vi "Write Configuration File from User.vi"(7 "Master?":bool=TRUE, 8 "error in":errorcluster, 10 "Master Config":T1 {"Conc Tolerance" min=0.0 max=100.0 step=1.0}, 11 "Test Config":T3={"Chopper RPM"=140, "IR Power"=5, "Conc Tolerance"=0.0, "Gas Stable Time"=0, "A-D Settle"=0, "Samples"=0, "Filter Time"=0, "Gas Mixtures"=[], "Filter Sequences"=[], "Functional Test"={"Mic Test ON ADC Max"=0.0, "Mic Test ON ADC Min"=0.0, "Mic Test OFF ADC Max"=0.0, "Mic Test OFF ADC Min"=0.0, "Mic Test IC ADC Max"=0.0, "Mic Test IC ADC Min"=0.0, "IR Emitter ON ADC Max"=0.0, "IR Emitter ON ADC Min"=0.0, "IR Emitter OFF ADC Max"=0.0, "IR Emitter OFF ADC Min"=0.0}, "Initial Flow Rate"=0.0, "Max Flow Rate"=0.0} {"Gas Mixtures"."ADC Gains" items=["0"=0, "3"=3, "4"=4, "5"=5, "6"=6, "7"=7]; "Conc Tolerance" min=0.0 max=100.0 step=1.0; "IR Power" min=2 max=5 step=1; "Chopper RPM" min=140 max=1000 step=1}) -> (0 "error out":errorcluster, 3 "Cancelled?":bool)   [LabVIEW 2015]
uses:
  Controls/Test Config.ctl
  Controls/Gas Mixture.ctl
  CAN Communication/PAS/Typedefs/ADC Gains.ctl
  Controls/Filter Sequence.ctl
  Controls/Functional Test.ctl
  Controls/Master Config.ctl
  Controls/Gas Info.ctl
  CAN Communication/PAS/PAS.lvclass
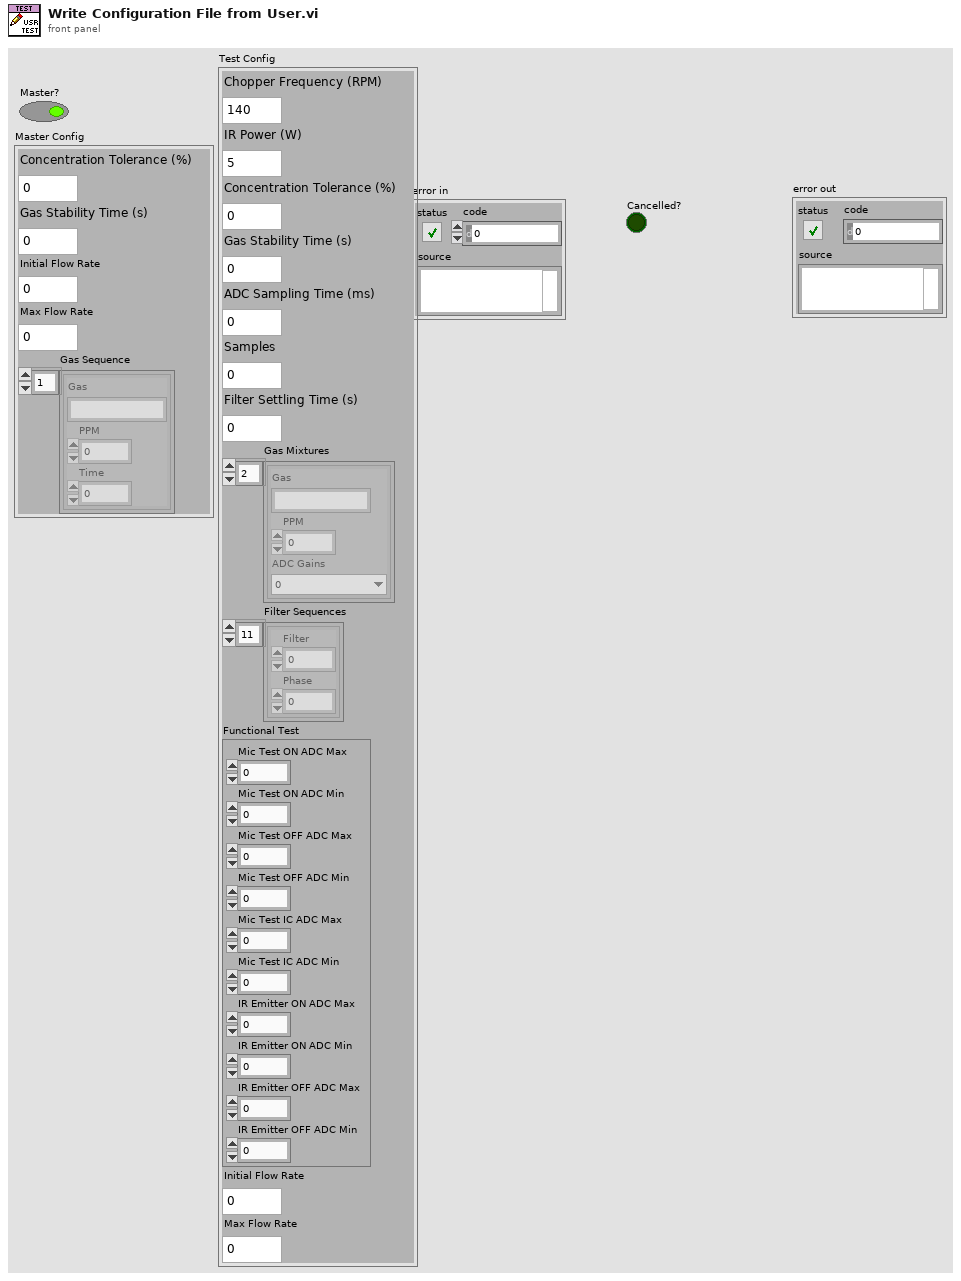
[diagram p1: front panel]
types:
  T1 = typedef "Master Config.ctl" = cluster{"Conc Tolerance":dbl, "Gas Stable Time":u16, "Initial Flow Rate":sgl, "Max Flow Rate":sgl, "Gas Sequence":T2[]}
  T2 = typedef "Gas Info.ctl" = cluster{"Gas":string, "PPM":dbl, "Time":u32}
  T3 = typedef "Test Config.ctl" = cluster{"Chopper RPM":u16, "IR Power":u8, "Conc Tolerance":dbl, "Gas Stable Time":u16, "A-D Settle":u16, "Samples":u16, "Filter Time":u16, "Gas Mixtures":T4[], "Filter Sequences":T6[], "Functional Test":T7, "Initial Flow Rate":sgl, "Max Flow Rate":sgl}
  T4 = typedef "Gas Mixture.ctl" = cluster{"Gas":string, "PPM":dbl, "ADC Gains":T5}
  T5 = typedef "PAS.lvclass/ADC Gains.ctl" = u16
  T6 = typedef "Filter Sequence.ctl" = cluster{"Filter":u8, "Phase":dbl}
  T7 = typedef "Functional Test.ctl" = cluster{"Mic Test ON ADC Max":dbl, "Mic Test ON ADC Min":dbl, "Mic Test OFF ADC Max":dbl, "Mic Test OFF ADC Min":dbl, "Mic Test IC ADC Max":dbl, "Mic Test IC ADC Min":dbl, "IR Emitter ON ADC Max":dbl, "IR Emitter ON ADC Min":dbl, "IR Emitter OFF ADC Max":dbl, "IR Emitter OFF ADC Min":dbl}
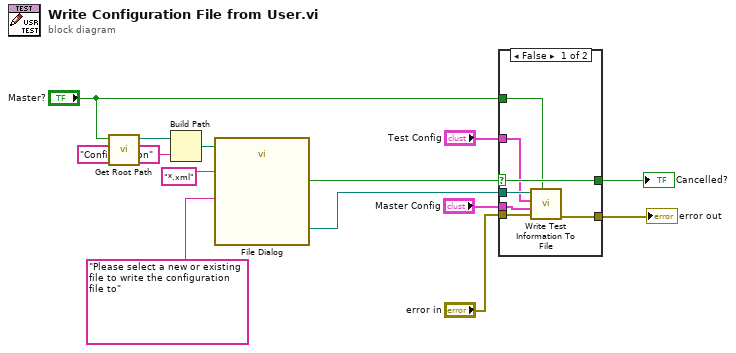
[diagram p0: block diagram]
diagram:
  n1 = call "Get Root Path.vi"("Master?"="Master?") -> ("Root Path"=w12:path)  [unwired: 10 in]
  n2 = Build Path(base path=w12, name or relative path="Configuration") -> (appended path=w11:path)
  n3 = call "File Dialog"("start path"=w11, "prompt"="Please select a new or existing file to write the configuration file to", "pattern (all files)"="*.xml") -> ("selected path"=w7:path, "cancelled"=w6:bool)  [unwired: 9 in, 2 out]
  n4 = case shown="False" w6 {
    selector: w6 -> [w17 w21]
    tunnel: "error in" -> [w20 w22]
    tunnel: [w19 w22] -> w8
    tunnel: w7 -> [w18 _]
    tunnel: [w17 w21] -> w5
    tunnel: "Test Config" -> [w16 _]
    tunnel: "Master?" -> [w14 _]
    tunnel: "Master Config" -> [w15 _]
    frame False {
      n5 = call "Write Test Information To File.vi"("Master?"=w14, "error in"=w20, "Master Config"=w15, "Test Config"=w16, "file path (use dialog)"=w18) -> ("error out"=w19:errorcluster)  [unwired: 6 in]
    }
    frame True {
    }
  }
  "error out" <- w8
  "Cancelled?" <- w5
